vi "svfa_Process Frequency Response (complex).vi"(0 "X FFT spectrum [Vrms]":cluster{"f0":dbl, "df":dbl, "spectrum":cdb[]} {"spectrum" format="%.2f"; "df" format="%.2f"; "f0" format="%.2f"}, 1 "processing control":T7(ring), 5 "spectrum info X":T1={"channel name"="", "description"="", "x-axis units"=0, "spectral info"={"spectrum type"=enum."Power [Magnitude^2]", "linear/dB"=enum."linear", "window"=0, "window size"=0, "FFT size"=0}, "engineering units"=0, "custom label"="", "dB reference [EU]"=0.0, "peak units"=enum."rms", "weighting filter"=0, "spectral density?"=FALSE, "unit label"="", "spectrum skewed?"=FALSE, "complimentary spectrum units"=enum."none"} {"x-axis units" items=["Time (s)"=0, "Frequency-CB (Hz)"=1, "Frequency-CPB (Hz)"=1248, "Frequency-Arbitrary (Hz)"=2357, "Quefrency (s)"=2, "Revolutions (rev)"=3, "Order"=4, "Speed (RPM)"=11, "Speed (rad/s)"=21, "Index"=65535]; "weighting filter" items=["Linear", "A-weighting", "B-weighting", "C-weighting", "ITU-R 468-4", "Dolby", "CCITT", "C-message", "Wb", "Wc", "Wd", "We", "Wf", "Wh", "Wj", "Wk", "Wm", "AES17 20 kHz lowpass", "AES17 40 kHz lowpass", "AES17 20 kHz highpass", "AES17 40 kHz highpass"]; "dB reference [EU]" format="%.2f"; "engineering units" items=["custom..."=0, "V"=1, "A"=21, "C"=30, "pC"=31, "s"=32, "-"=29, "Pa"=2, "N"=20, "g"=3, "m/s^2"=4, "m/s"=5, "m"=6, "mm/s"=12, "mm"=13, "micron/s"=14, "micron"=15, "in/s^2"=7, "in/s"=8, "in"=9, "mil/s"=10, "mil"=11, "rad/s^2"=16, "rad/s"=17, "rad"=18, "deg/s^2"=26, "deg/s"=27, "deg"=28, "RPM"=22, "cycle/s^2"=23, "Hz"=24, "cycle"=25, "strain"=19]; "spectral info"."window" items=["None "=0, "Hanning"=1, "Hamming"=2, "Blackman-Harris"=3, "Exact Blackman"=4, "Blackman"=5, "Flat Top"=6, "4 Term B-Harris "=7, "7 Term B-Harris"=8, "Low Sidelobe"=9, "Force - Exponential"=10, "Gaussian"=62]}, 7 "Y FFT spectrum [Vrms]":cluster{"f0":dbl, "df":dbl, "spectrum":cdb[]} {"spectrum" format="%.2f"; "df" format="%.2f"; "f0" format="%.2f"}, 9 "spectrum info Y":T1={"channel name"="", "description"="", "x-axis units"=0, "spectral info"={"spectrum type"=enum."Power [Magnitude^2]", "linear/dB"=enum."linear", "window"=0, "window size"=0, "FFT size"=0}, "engineering units"=0, "custom label"="", "dB reference [EU]"=0.0, "peak units"=enum."rms", "weighting filter"=0, "spectral density?"=FALSE, "unit label"="", "spectrum skewed?"=FALSE, "complimentary spectrum units"=enum."none"} {"x-axis units" items=["Time (s)"=0, "Frequency-CB (Hz)"=1, "Frequency-CPB (Hz)"=1248, "Frequency-Arbitrary (Hz)"=2357, "Quefrency (s)"=2, "Revolutions (rev)"=3, "Order"=4, "Speed (RPM)"=11, "Speed (rad/s)"=21, "Index"=65535]; "weighting filter" items=["Linear", "A-weighting", "B-weighting", "C-weighting", "ITU-R 468-4", "Dolby", "CCITT", "C-message", "Wb", "Wc", "Wd", "We", "Wf", "Wh", "Wj", "Wk", "Wm", "AES17 20 kHz lowpass", "AES17 40 kHz lowpass", "AES17 20 kHz highpass", "AES17 40 kHz highpass"]; "dB reference [EU]" format="%.2f"; "engineering units" items=["custom..."=0, "V"=1, "A"=21, "C"=30, "pC"=31, "s"=32, "-"=29, "Pa"=2, "N"=20, "g"=3, "m/s^2"=4, "m/s"=5, "m"=6, "mm/s"=12, "mm"=13, "micron/s"=14, "micron"=15, "in/s^2"=7, "in/s"=8, "in"=9, "mil/s"=10, "mil"=11, "rad/s^2"=16, "rad/s"=17, "rad"=18, "deg/s^2"=26, "deg/s"=27, "deg"=28, "RPM"=22, "cycle/s^2"=23, "Hz"=24, "cycle"=25, "strain"=19]; "spectral info"."window" items=["None "=0, "Hanning"=1, "Hamming"=2, "Blackman-Harris"=3, "Exact Blackman"=4, "Blackman"=5, "Flat Top"=6, "4 Term B-Harris "=7, "7 Term B-Harris"=8, "Low Sidelobe"=9, "Force - Exponential"=10, "Gaussian"=62]}, 11 "error in (no error)":errorcluster, 12 "averaging parameters":T8={"averaging mode"=enum."No averaging", "weighting mode"=enum."Linear", "number of averages"=10, "linear mode"=enum."Auto restart"}, 13 "FRF mode":enum16{"H1", "H2", "H3"}(ring)) -> (3 "averaging done":bool, 4 "complex spectrum":T9={"f0"=0.0, "df"=1.0, "complex spectrum"=[]} {"complex spectrum" format="%.2f"; "df" format="%.2f"; "f0" format="%.2f"}, 8 "coherence":cluster{"f0":dbl, "df":dbl, "spectrum":dbl[]} {"spectrum" format="%.2f"; "df" format="%.2f"; "f0" format="%.2f"}, 10 "spectrum info":T1={"channel name"="", "description"="", "x-axis units"=0, "spectral info"={"spectrum type"=enum."Power [Magnitude^2]", "linear/dB"=enum."linear", "window"=0, "window size"=0, "FFT size"=0}, "engineering units"=0, "custom label"="", "dB reference [EU]"=0.0, "peak units"=enum."rms", "weighting filter"=0, "spectral density?"=FALSE, "unit label"="", "spectrum skewed?"=FALSE, "complimentary spectrum units"=enum."none"} {"x-axis units" items=["Time (s)"=0, "Frequency-CB (Hz)"=1, "Frequency-CPB (Hz)"=1248, "Frequency-Arbitrary (Hz)"=2357, "Quefrency (s)"=2, "Revolutions (rev)"=3, "Order"=4, "Speed (RPM)"=11, "Speed (rad/s)"=21, "Index"=65535]; "weighting filter" items=["Linear", "A-weighting", "B-weighting", "C-weighting", "ITU-R 468-4", "Dolby", "CCITT", "C-message", "Wb", "Wc", "Wd", "We", "Wf", "Wh", "Wj", "Wk", "Wm", "AES17 20 kHz lowpass", "AES17 40 kHz lowpass", "AES17 20 kHz highpass", "AES17 40 kHz highpass"]; "dB reference [EU]" format="%.2f"; "engineering units" items=["custom..."=0, "V"=1, "A"=21, "C"=30, "pC"=31, "s"=32, "-"=29, "Pa"=2, "N"=20, "g"=3, "m/s^2"=4, "m/s"=5, "m"=6, "mm/s"=12, "mm"=13, "micron/s"=14, "micron"=15, "in/s^2"=7, "in/s"=8, "in"=9, "mil/s"=10, "mil"=11, "rad/s^2"=16, "rad/s"=17, "rad"=18, "deg/s^2"=26, "deg/s"=27, "deg"=28, "RPM"=22, "cycle/s^2"=23, "Hz"=24, "cycle"=25, "strain"=19]; "spectral info"."window" items=["None "=0, "Hanning"=1, "Hamming"=2, "Blackman-Harris"=3, "Exact Blackman"=4, "Blackman"=5, "Flat Top"=6, "4 Term B-Harris "=7, "7 Term B-Harris"=8, "Low Sidelobe"=9, "Force - Exponential"=10, "Gaussian"=62]}, 14 "averages completed":dbl format="%.2f", 15 "error out":errorcluster)   [LabVIEW 2017]
uses:
  <vilib>/addons/_NISVFA/_Shared subVIs/Controls/svc_Spectrum Info.ctl
  <vilib>/addons/_NISVFA/_Shared subVIs/Controls/svc_X-Axis Units.ctl
  <vilib>/addons/_NISVFA/_Shared subVIs/Controls/svc_Spectrum Type.ctl
  <vilib>/addons/_NISVFA/_Shared subVIs/Controls/svc_Engineering Units Text Ring.ctl
  <vilib>/addons/_NISVFA/_Shared subVIs/Controls/svc_Weighting Filter Text Ring.ctl
  <vilib>/addons/_NISVFA/_Shared subVIs/Controls/svc_Complimentary Spectrum Units.ctl
  <vilib>/addons/_NISVFA/_Shared subVIs/Spectrum Averaging/svfa_Average Spectrum (complex) No State.vi
  <vilib>/addons/_NISVFA/_Shared subVIs/Spectrum Averaging/svfa_Reset Averaging State Info.vi
  <vilib>/addons/_NISVFA/_Shared subVIs/Spectrum Averaging/svfa_Average Array with Avg Checks (complex) No State.vi
  <vilib>/addons/_NISVFA/_Shared subVIs/Spectrum Averaging/svfa_Average Array (complex) No State.vi
  <vilib>/addons/_NISVFA/_Shared subVIs/Spectrum Averaging/svfa_No Average Array (complex).vi
  <vilib>/addons/_NISVFA/_Shared subVIs/Spectrum Averaging/svfa_Average Array (complex).vi
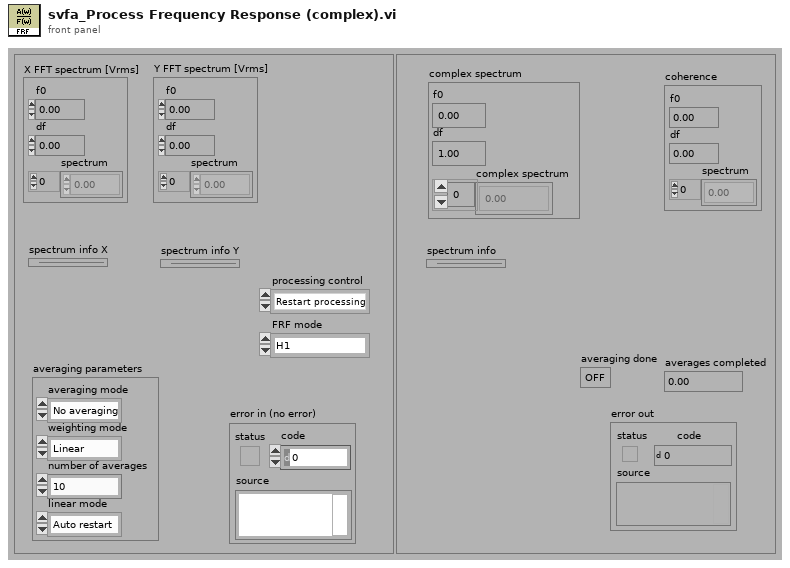
[diagram p1: front panel]
types:
  T1 = typedef "svc_Spectrum Info.ctl" = cluster{"channel name":string, "description":string, "x-axis units":T2, "spectral info":cluster{"spectrum type":T3, "linear/dB":enum16{"linear", "dB"}, "window":u16, "window size":i32, "FFT size":i32}, "engineering units":T4, "custom label":string, "dB reference [EU]":dbl, "peak units":enum16{"rms", "peak", "peak-peak"}, "weighting filter":T5, "spectral density?":bool, "unit label":string, "spectrum skewed?":bool, "complimentary spectrum units":T6}
  T2 = typedef "svc_X-Axis Units.ctl" = u16
  T3 = typedef "svc_Spectrum Type.ctl" = enum16{"FFT Spectrum [complex]", "Amplitude [Magnitude]", "Power [Magnitude^2]", "Cross Spectrum [complex]", "Frequency Response [Complex]"}
  T4 = typedef "svc_Engineering Units Text Ring.ctl" = u16
  T5 = typedef "svc_Weighting Filter Text Ring.ctl" = u16
  T6 = typedef "svc_Complimentary Spectrum Units.ctl" = enum16{"none", "radians", "degrees", "cycles", "imaginary"}
  T7 = enum16{"Restart processing", "Continue processing", "Skip processing"}
  T8 = cluster{"averaging mode":enum16{"No averaging", "Vector averaging", "RMS averaging", "Peak hold"}, "weighting mode":enum16{"Linear", "Exponential"}, "number of averages":u32, "linear mode":enum16{"One shot", "Auto restart"}}
  T9 = cluster{"f0":dbl, "df":dbl, "complex spectrum":cdb[]}
  T10 = enum16{"No averaging", "Vector averaging", "RMS averaging", "Peak hold"}
  T11 = cluster{"complex spectrum":cluster{"f0":dbl, "df":dbl, "complex spectrum":cdb[]}, "spectrum info":T1}
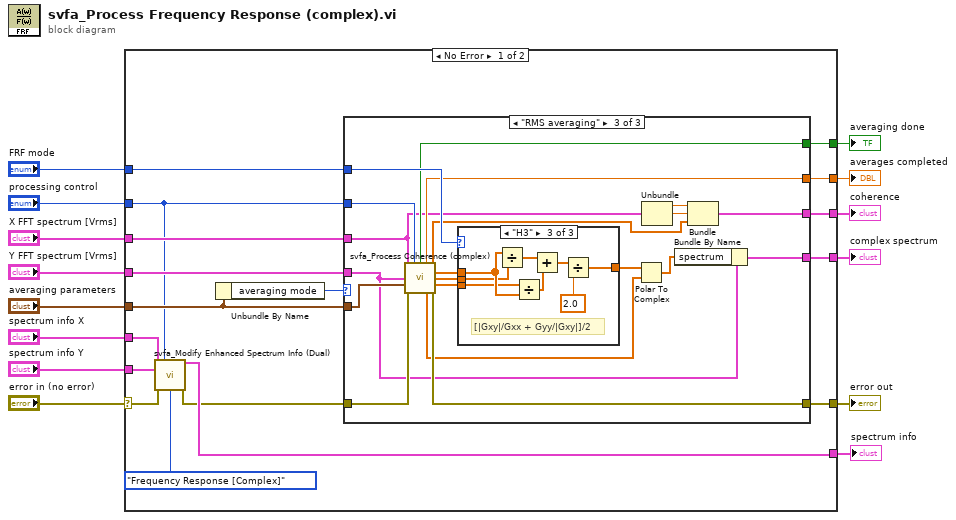
[diagram p0: block diagram]
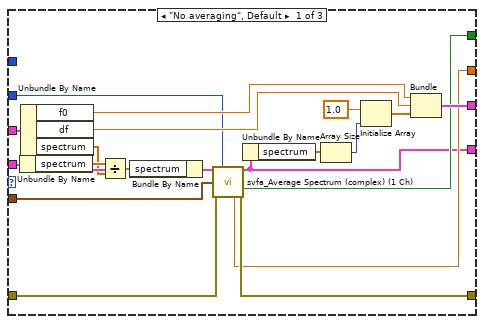
[diagram p2: hidden frame]
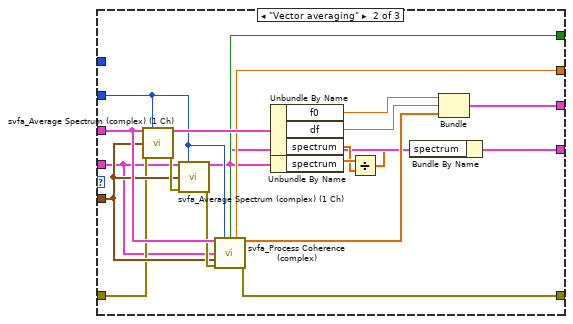
[diagram p3: hidden frame]
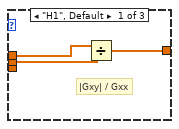
[diagram p4: hidden frame]
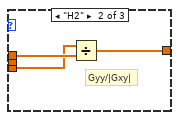
[diagram p5: hidden frame]
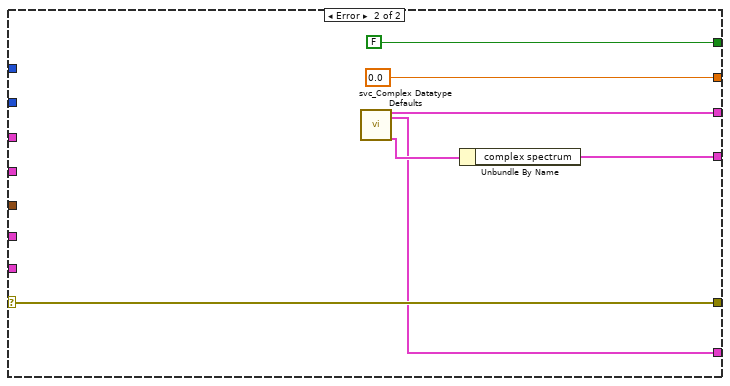
[diagram p6: hidden frame]
diagram:
  n1 = case shown="No Error" "error in (no error)" {
    selector: "error in (no error)" -> [w28 w112]
    tunnel: "Y FFT spectrum [Vrms]" -> [w31 _]
    tunnel: "X FFT spectrum [Vrms]" -> [w22 _]
    tunnel: [w16 w107] -> w12
    tunnel: [w17 w109] -> w11
    tunnel: [w24 FALSE ("averaging done")] -> w10
    tunnel: "averaging parameters" -> [w30 _]
    tunnel: [w29 w112] -> w8
    tunnel: "spectrum info X" -> [w27 _]
    tunnel: "spectrum info Y" -> [w26 _]
    tunnel: "FRF mode" -> [w25 _]
    tunnel: [w23 0.0 ("averages completed")] -> w3
    tunnel: "processing control" -> [w15 _]
    tunnel: [w21 w106] -> w1
    frame No Error {
      n2 = call <vilib>:"svfa_Modify Enhanced Spectrum Info (Dual).vi"("spectrum info X"=w27, "processing control"=w15, "spectrum info Y"=w26, "error in (no error)"=w28, "spectrum type"=svc_Spectrum_Type."Frequency Response [Complex]") -> ("spectrum info"=w21:T1, "error out"=w19:errorcluster)  [unwired: 8 in, 1 out]
      n3 = Unbundle By Name(w30) -> ("averaging mode"=w20:T10)
      n4 = case shown="\"RMS averaging\"" w20 {
        tunnel: [w34 w52 w78] -> w16
        tunnel: [w44 w64 w89] -> w29
        tunnel: w30 -> [w37 w62 w88]
        tunnel: [w39 w67 w86] -> w24
        tunnel: w22 -> [w50 w70 w76]
        tunnel: w31 -> [w47 w59 w79]
        tunnel: w19 -> [w45 w61 w90]
        tunnel: w25 -> [_ _ w87]
        tunnel: [w38 w66 w85] -> w23
        tunnel: w15 -> [w36 w60 w84]
        tunnel: [w40 w57 w73] -> w17
        frame "No averaging", Default {
          n5 = Unbundle By Name(w47) -> ("spectrum"=w51:cdb[])
          n6 = Unbundle By Name(w50) -> ("f0"=w41:dbl, "df"=w42:dbl, "spectrum"=w35:cdb[])
          n7 = Divide(x=w51, y=w35) -> (x/y=w48:cdb[])
          n8 = Bundle By Name(cluster=w47, "spectrum"=w48) -> (w46:cluster{"f0":dbl, "df":dbl, "spectrum":cdb[]})
          n9 = call <vilib>:"svfa_Average Spectrum (complex) (1 Ch).vi"("spectrum"=w46, "processing control"=w36, "averaging parameters"=w37, "error in (no error)"=w45) -> ("spectrum"=w34:cluster{"f0":dbl, "df":dbl, "spectrum":cdb[]}, "averaging done"=w39:bool, "averages completed"=w38:dbl, "error out"=w44:errorcluster)  [unwired: 7 in, 1 out]
          n10 = Unbundle By Name(w34) -> ("spectrum"=w33:cdb[])
          n11 = Array Size(array=w33) -> (size(s)=w32:i32)
          n12 = Initialize Array(1.0 ("overwrite value"), w32) -> (w43:dbl[])
          n13 = Bundle("f0"=w41, "df"=w42, w43) -> (w40:cluster{"f0":dbl, "df":dbl, dbl[]})  [unwired: 1 in]
        }
        frame "Vector averaging" {
          n14 = call <vilib>:"svfa_Average Spectrum (complex) (1 Ch).vi"("spectrum"=w70, "processing control"=w60, "averaging parameters"=w62, "error in (no error)"=w61) -> ("spectrum"=w69:cluster{"f0":dbl, "df":dbl, "spectrum":cdb[]}, "error out"=w68:errorcluster)  [unwired: 7 in, 3 out]
          n15 = call <vilib>:"svfa_Average Spectrum (complex) (1 Ch).vi"("spectrum"=w59, "processing control"=w60, "averaging parameters"=w62, "error in (no error)"=w68) -> ("spectrum"=w54:cluster{"f0":dbl, "df":dbl, "spectrum":cdb[]}, "error out"=w65:errorcluster)  [unwired: 7 in, 3 out]
          n16 = call <vilib>:"svfa_Process Coherence (complex).vi"("X FFT spectrum [Vrms]"=w70, "processing control"=w60, "Y FFT spectrum [Vrms]"=w59, "averaging parameters"=w62, "error in (no error)"=w65) -> ("averaging done"=w67:bool, "averages completed"=w66:dbl, "Coherence"=w58:dbl[], "error out"=w64:errorcluster)  [unwired: 3 in, 4 out]
          n17 = Unbundle By Name(w69) -> ("f0"=w55:dbl, "df"=w56:dbl, "spectrum"=w63:cdb[])
          n18 = Unbundle By Name(w54) -> ("spectrum"=w71:cdb[])
          n19 = Divide(x=w71, y=w63) -> (x/y=w53:cdb[])
          n20 = Bundle By Name(cluster=w54, "spectrum"=w53) -> (w52:cluster{"f0":dbl, "df":dbl, "spectrum":cdb[]})
          n21 = Bundle("f0"=w55, "df"=w56, "Coherence"=w58) -> (w57:cluster{"f0":dbl, "df":dbl, "Coherence":dbl[]})  [unwired: 1 in]
        }
        frame "RMS averaging" {
          n22 = call <vilib>:"svfa_Process Coherence (complex).vi"("X FFT spectrum [Vrms]"=w76, "processing control"=w84, "Y FFT spectrum [Vrms]"=w79, "averaging parameters"=w88, "error in (no error)"=w90) -> ("averaging done"=w86:bool, "averages completed"=w85:dbl, "Coherence"=w72:dbl[], "MAG <Gxy>"=w82:dbl[], "<Gxx>"=w81:dbl[], "<Gyy>"=w80:dbl[], "PHASE <Gxy>"=w83:dbl[], "error out"=w89:errorcluster)  [unwired: 3 in]
          n23 = case shown="\"H3\"" w87 {
            tunnel: w80 -> [_ w95 w98]
            tunnel: [w94 w97 w105] -> w91
            tunnel: w81 -> [w92 _ w99]
            tunnel: w82 -> [w93 w96 w100]
            frame "H1", Default {
              # "|Gxy| / Gxx"
              n24 = Divide(x=w93, y=w92) -> (x/y=w94:dbl[])
            }
            frame "H2" {
              # "Gyy/|Gxy|"
              n25 = Divide(x=w95, y=w96) -> (x/y=w97:dbl[])
            }
            frame "H3" {
              # "[|Gxy|/Gxx + Gyy/|Gxy|]/2"
              n26 = Divide(x=w100, y=w99) -> (x/y=w101:dbl[])
              n27 = Divide(x=w98, y=w100) -> (x/y=w102:dbl[])
              n28 = Add(x=w101, y=w102) -> (x+y=w103:dbl[])
              n29 = Divide(x=w103, y=2.0) -> (x/y=w105:dbl[])
            }
          }
          n30 = Polar To Complex(1:w83, 2:w91) -> (0:w77:cdb[])
          n31 = Unbundle(w76) -> ("f0"=w75:dbl, "df"=w74:dbl)  [unwired: 1 out]
          n32 = Bundle By Name(cluster=w79, "spectrum"=w77) -> (w78:cluster{"f0":dbl, "df":dbl, "spectrum":cdb[]})
          n33 = Bundle("f0"=w75, "df"=w74, "Coherence"=w72) -> (w73:cluster{"f0":dbl, "df":dbl, "Coherence":dbl[]})  [unwired: 1 in]
        }
      }
    }
    frame Error {
      n34 = call <vilib>:"svc_Complex Datatype Defaults.vi"() -> ("empty spectrum"=w109:cluster{"f0":dbl, "df":dbl, "magnitude":dbl[]}, "dead spectrum info"=w106:T1, "complex spectrum"=w108:T11)  [unwired: 11 in, 6 out]
      n35 = Unbundle By Name(w108) -> ("complex spectrum"=w107:T9)
    }
  }
  "complex spectrum" <- w12
  "coherence" <- w11
  "averaging done" <- w10
  "averages completed" <- w3
  "error out" <- w8
  "spectrum info" <- w1
